vi "Test Cashier Place Order.vi"(8 "error in (no error)":errorcluster, 11 "Cashier Test in":refnum<class "Cashier Test.lvclass">) -> (0 "error out":errorcluster, 3 "Cashier Test out":refnum<class "Cashier Test.lvclass">)   [LabVIEW 2020, in "Cashier Test.lvclass"]
uses:
  Cashier Test.lvclass
  C:/Program Files (x86)/National Instruments/LabVIEW 2020/vi.lib/Asteme/LUnit/Test Case.lvclass
  Mock Worker/Mock Job Processor.lvclass
  C:/Users/anton/Documents/GitHub/Triarc-Examples/Coffee Shop/Process Job/Job Handler.lvclass
  Cashier/Cashier.lvclass
  C:/Users/anton/Documents/GitHub/Triarc-Examples/Coffee Shop/Worker/Worker.lvclass
  C:/Program Files (x86)/National Instruments/LabVIEW 2020/vi.lib/Asteme/Triarc Framework/Process/Process.lvclass
  Support/Beverages/TypeDefs/Drink Type.ctl
  Support/Beverages/TypeDefs/Options.ctl
  Customer/Customer.lvclass
  <vilib>/Asteme/Triarc Framework/Process/Process.lvclass/Process.ctl
  <vilib>/Asteme/LUnit/Test Case.lvclass/Test Case.ctl
  <vilib>/Asteme/LUnit/LUnit Assertion Result.lvclass/LUnit Assertion Result.ctl
  <vilib>/Asteme/Triarc Framework/Process/Private/SubVIs/Wait for finish.vi
  <vilib>/Asteme/Triarc Framework/Process/Protected/Messaging/Enqueue Message.vi
  <vilib>/Asteme/Triarc Framework/Process/Private/SubVIs/Set Lifecycle State.vi
  <vilib>/Asteme/Triarc Framework/Process/Public/Lifecycle/Get Lifecycle State.vi
  <vilib>/Asteme/LUnit/Palette/Fail.vi
  <vilib>/Asteme/LUnit/Palette/Pass.vi
  <vilib>/Asteme/LUnit/Set Assertion Type.vi
  <vilib>/Utility/error.llb/Clear Errors.vi
  <vilib>/Asteme/LUnit/Add test result.vi
  <vilib>/Asteme/LUnit/LUnit Write Passed.vi
  <vilib>/Asteme/LUnit/LUnit Get Test Case.vi
  <vilib>/Asteme/LUnit/Assertion Result/LUnit Get Test Name.vi
  <vilib>/Asteme/LUnit/LUnit Write Message.vi
  <vilib>/Asteme/LUnit/LUnit Write Description.vi
  <vilib>/Asteme/LUnit/LUnit Write Assertion Type.vi
  <vilib>/Asteme/LUnit/Read Test Case Name.vi
  <vilib>/Utility/error.llb/Error Cluster From Error Code.vi
  <vilib>/Asteme/LUnit/LUnit Assertion Result.lvclass
  Support/Order/Order.lvclass
  <vilib>/Asteme/Triarc Framework/Process/Process.lvclass
  Worker/Worker.lvclass
  <vilib>/Asteme/LUnit/Test Case.lvclass
  Support/Beverages/Beverage/Beverage.lvclass
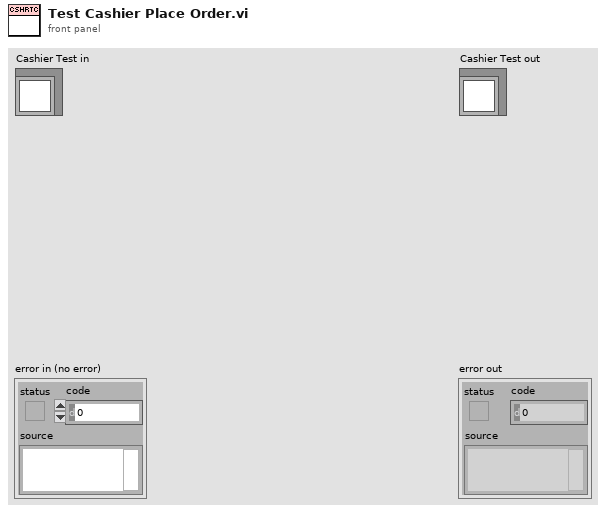
[diagram p1: front panel]
types:
  T1 = typedef "Beverage.lvclass/Drink Type.ctl" = enum16{"Dark Roast", "Decaf", "Espresso", "House Blend"}
  T2 = typedef "Beverage.lvclass/Options.ctl" = enum16{"<None>", "Milk", "Mocha", "Soy", "Whip"}
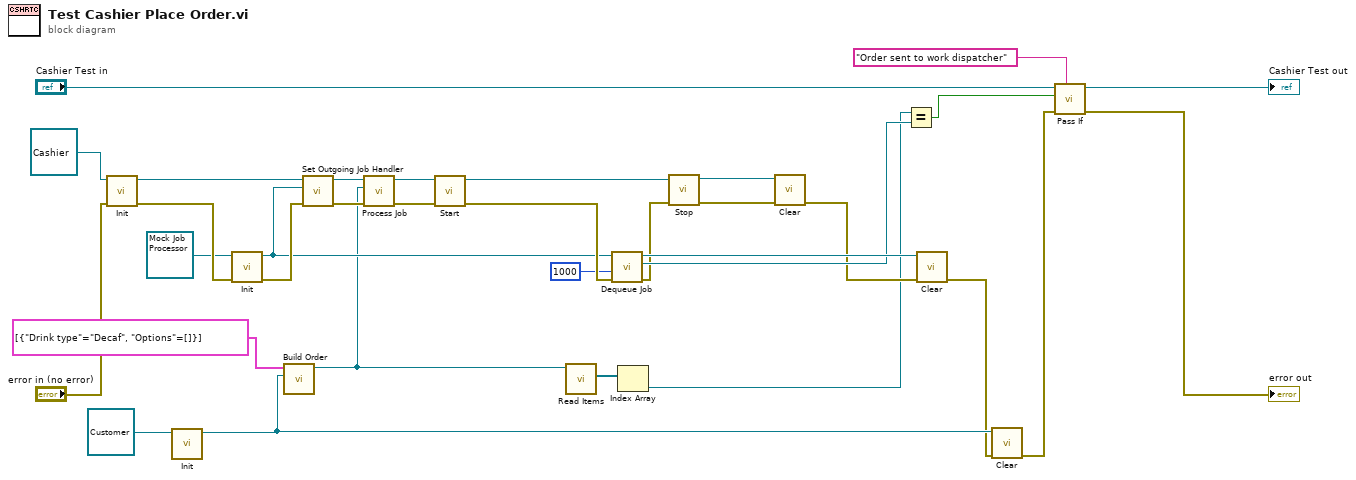
[diagram p0: block diagram]
diagram:
  n1 = call-dynamic "Init.vi"("error in (no error)"="error in (no error)", "View In"=refnum<class "Cashier.lvclass"> refnum ("Cashier.lvclass")) -> ("error out"=w32:errorcluster, "View Out"=w33:refnum<class "Cashier.lvclass">)  [unwired: 8 in]
  n2 = call-dynamic "Init.vi"("View In"=refnum<class "Customer.lvclass"> refnum ("Customer.lvclass")) -> ("View Out"=w6:refnum<class "Customer.lvclass">)  [unwired: 9 in, 1 out]
  n3 = call-dynamic "Init.vi"("error in (no error)"=w32, "Mock Worker In"=refnum<class "Mock Job Processor.lvclass"> refnum) -> ("error out"=w25:errorcluster, "Mock Worker Out"=w14:refnum<class "Mock Job Processor.lvclass">)  [unwired: 8 in]
  n4 = call "Build Order.vi"("Customer"=w6, "Order"=cluster{"Drink type":T1, "Options":T2[]}[] [{"Drink type"=enum."Decaf", "Options"=[]}]) -> ("Order Out"=w3:refnum<class "Order.lvclass">)  [unwired: 7 in, 2 out]
  n5 = call "Set Outgoing Job Handler.vi"("error in (no error)"=w25, "Work Dispatcher"=w14, "Worker In"=w33) -> ("error out"=w23:errorcluster, "Worker Out"=w24:refnum<class "Cashier.lvclass">)  [unwired: 7 in]
  n6 = call-dynamic "Process Job.vi"("error in (no error)"=w23, "Task"=w3, "Worker In"=w24) -> ("error out"=w21:errorcluster, "Worker Out"=w22:refnum<class "Cashier.lvclass">)  [unwired: 7 in]
  n7 = call <vilib>:"Start.vi"("error in (no error)"=w21, "Process In"=w22) -> ("error out"=w26:errorcluster, "Process Out"=w31:refnum<class "Cashier.lvclass">)  [unwired: 8 in]
  n8 = call-dynamic "Read Items.vi"("Order in"=w3) -> ("Items"=w2:refnum<class "Beverage.lvclass">[])  [unwired: 8 in, 2 out]
  n9 = call "Dequeue Job.vi"("error in (no error)"=w26, "timeout in ms (-1)"=1000, "Mock Worker in"=w14) -> ("error out"=w18:errorcluster, "element"=w20:refnum<class>, "Mock Worker out"=w27:refnum<class "Mock Job Processor.lvclass">)  [unwired: 5 in, 1 out]
  n10 = Index Array(array=w2) -> (element=w1:refnum<class "Beverage.lvclass">)  [unwired: 1 in]
  n11 = call <vilib>:"Stop.vi"("error in (no error)"=w18, "Process In"=w31) -> ("error out"=w29:errorcluster, "Process Out"=w30:refnum<class "Cashier.lvclass">)  [unwired: 7 in, 1 out]
  n12 = call-dynamic "Clear.vi"("error in (no error)"=w29, "View In"=w30) -> ("error out"=w17:errorcluster)  [unwired: 9 in]
  n13 = Equal?(x=w1, y=w20) -> (x = y?=w10:bool)
  n14 = call-dynamic "Clear.vi"("error in (no error)"=w17, "Mock Worker In"=w27) -> ("error out"=w5:errorcluster)  [unwired: 9 in]
  n15 = call-dynamic "Clear.vi"("error in (no error)"=w5, "View In"=w6) -> ("error out"=w4:errorcluster)  [unwired: 9 in]
  n16 = call <vilib>:"Pass If.vi"("Description"="Order sent to work dispatcher", "error in (no error)"=w4, "Pass?"=w10, "Test Case In"="Cashier Test in") -> ("error out"=→"error out":errorcluster, "Test Case Out"=→"Cashier Test out":refnum<class "Cashier Test.lvclass">)  [unwired: 6 in]
